vi "Destroy User Events.vi"(11 "UI Template in":refnum<class "Root.lvclass">) -> (3 "UI Template out":refnum<class "Root.lvclass">)   [LabVIEW 2025, in "Root.lvlib" / "Root.lvclass"]
uses:
  Root.lvclass
  Root.lvclass/Root.ctl
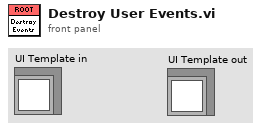
[diagram p1: front panel]
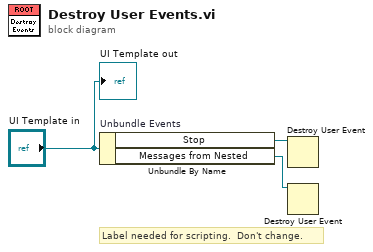
[diagram p0: block diagram]
diagram:
  # "Label needed for scripting.  Don't change."
  n1 = Unbundle By Name "Unbundle Events"("UI Template in") -> ("Stop"=w2:refnum<user-event>, "Messages from Nested"=w1:refnum<user-event>)
  n2 = Destroy User Event(user event=w2) -> ()  [unwired: 1 in, 1 out]
  n3 = Destroy User Event(user event=w1) -> ()  [unwired: 1 in, 1 out]
  "UI Template out" <- "UI Template in"
